vi "Switch On Button Press With Override.vi"(1 "Override False":bool, 2 "Button":bool, 3 "Override True":bool) -> (0 "Output":bool)   [LabVIEW 2018]
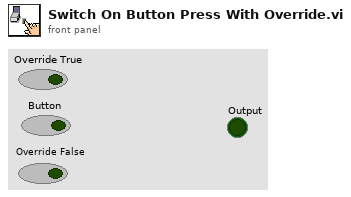
[diagram p1: front panel]
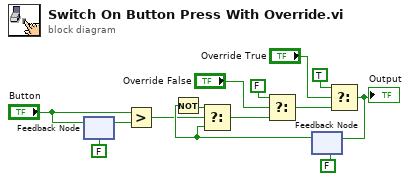
[diagram p0: block diagram]
diagram:
  n1 = feedback #1(FALSE ("Button")) -> (w10:bool)
  n2 = feedback-in #1("Button") -> ()
  n3 = Greater?(x="Button", y=w10) -> (0:w12:bool)
  n4 = feedback #2(FALSE) -> (w14:bool)
  n5 = Not(x=w14) -> (.not. x?=w13:bool)
  n6 = Select(t=w13, s=w12, f=w14) -> (s? t:f=w7:bool)
  n7 = Select(t=FALSE, s="Override False", f=w7) -> (s? t:f=w6:bool)
  n8 = Select(t=TRUE, s="Override True", f=w6) -> (s? t:f=w2:bool)
  "Output" <- w2
  n9 = feedback-in #2(w2) -> ()
